vi "Test 5.vi"(8 "error in (no error)":errorcluster, 11 "Test Case In":refnum<class "Tests.lvclass">) -> (0 "error out":errorcluster, 3 "Test Case Out":refnum<class "Tests.lvclass">)   [LabVIEW 2021, in "Tests.lvclass"]
uses:
  Tests.lvclass
  Tests.lvclass/Tests.ctl
  4993e8ee-a06a-463a-9684-69129f64d5ce.vi
  Proto/Module.lvclass
  edd98eef-76eb-44a5-86a1-b5d8b1cbf7a6.vi
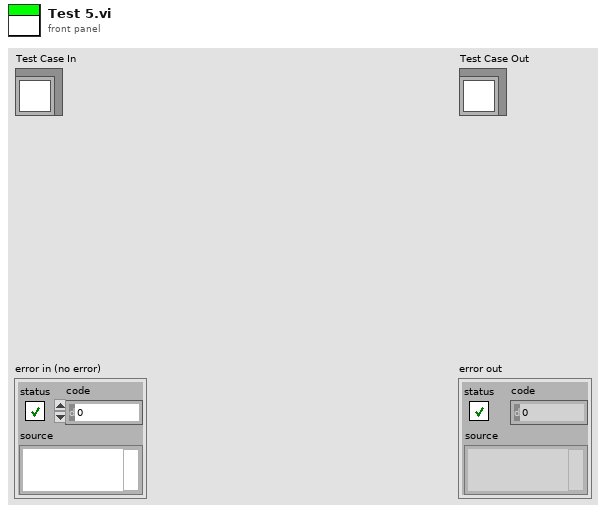
[diagram p1: front panel]
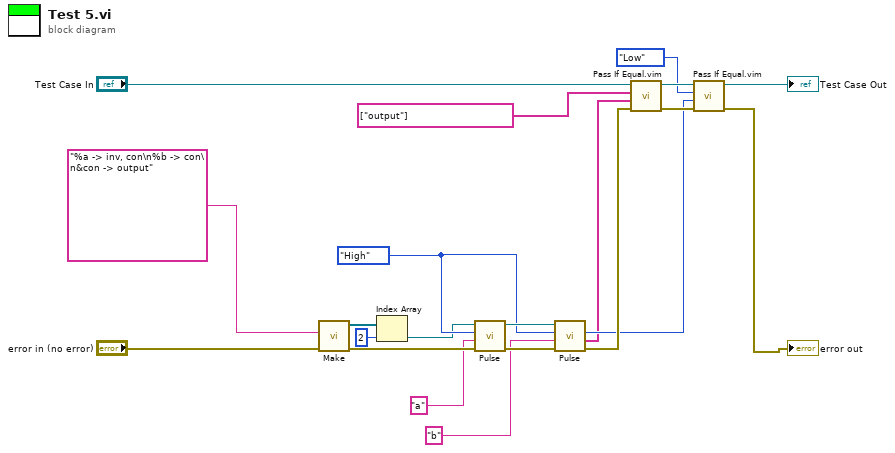
[diagram p0: block diagram]
diagram:
  w7 = enum16{"Low", "High"}."High" ("Pulse In")
  n1 = call "Make.vi"("error in (no error)"="error in (no error)", "Input"="%a -> inv, con\n%b -> con\n&con -> output") -> ("error out"=w18:errorcluster, "Proto"=w16:refnum<class "Module.lvclass">[])  [unwired: 8 in]
  n2 = Index Array(array=w16, index=2) -> (element=w4:refnum<class "Module.lvclass">)
  n3 = call-dynamic "Pulse.vi"("error in (no error)"=w18, "Sender"="a", "Pulse In"=w7, "Module In"=w4) -> ("error out"=w17:errorcluster, "Module Out"=w8:refnum<class "Module.lvclass">)  [unwired: 4 in, 2 out]
  n4 = call-dynamic "Pulse.vi"("error in (no error)"=w17, "Sender"="b", "Pulse In"=w7, "Module In"=w8) -> ("error out"=w9:errorcluster, "Receivers"=w5:string[], "Pulse Out"=w6:enum16{"Low", "High"})  [unwired: 4 in, 1 out]
  n5 = call "Pass If Equal.vim"("error in (no error)"=w9, "Actual"=w5, "Expected"=string[] ["output"] ("Receivers"), "LUnit Test Case In"="Test Case In") -> ("error out"=w19:errorcluster, "LUnit Test Case Out"=w12:refnum<class "Tests.lvclass">)  [unwired: 6 in]
  n6 = call "Pass If Equal.vim"("error in (no error)"=w19, "Actual"=w6, "Expected"=enum16{"Low", "High"}."Low" ("Pulse In"), "LUnit Test Case In"=w12) -> ("error out"=→"error out":errorcluster, "LUnit Test Case Out"=→"Test Case Out":refnum<class "Tests.lvclass">)  [unwired: 6 in]
